vi "find frequency.vi"(9 "target frequency":dbl format="%.2f") -> (1 "Min":bool, 2 "Max":bool, 3 "ClockDivisor":i32, 4 "Frequency":dbl format="%.2f", 5 "FreqDivisor":i32, 6 "Clock Source":string)   [LabVIEW 2021]
panel:
  out "MinimumFreqOut freq at 48 MHz":dbl format="%.2f"
  out "Minimum FreqOut freq at 750k":dbl format="%.2f"
  in  "value, factor1, factor2":i32[][](array[numeric])=array65536x3[196608 elements]
  # "constant array of values"
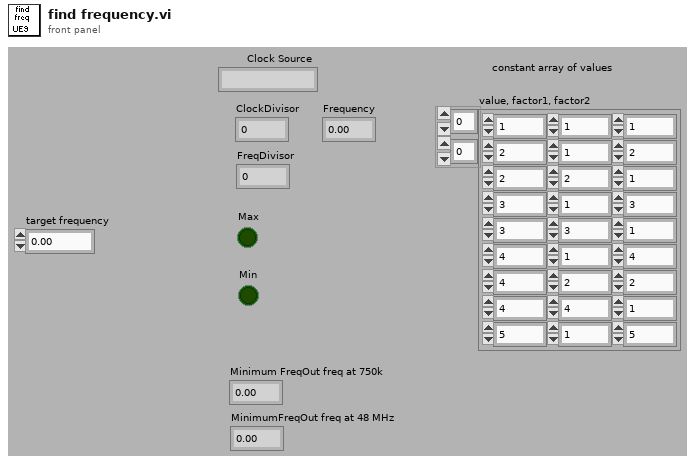
[diagram p1: front panel]
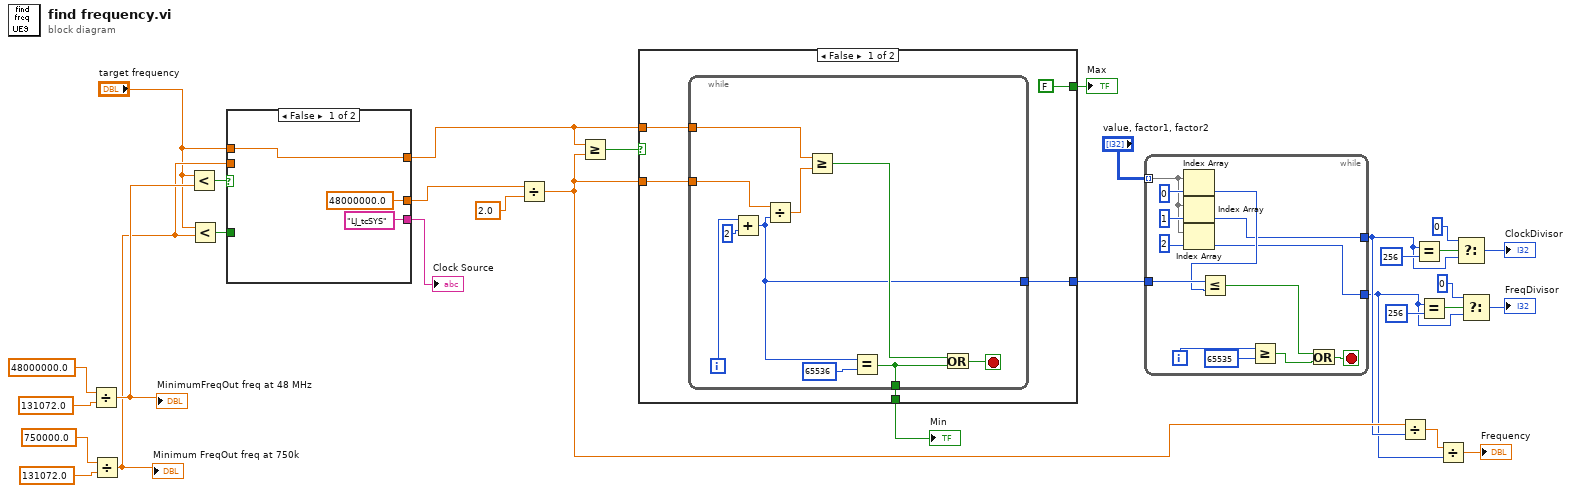
[diagram p0: block diagram]
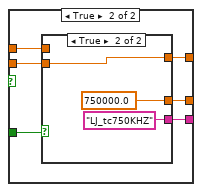
[diagram p2: hidden frame]
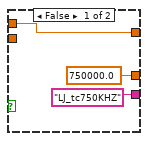
[diagram p3: hidden frame]
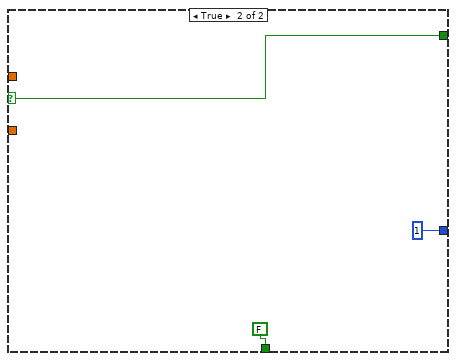
[diagram p4: hidden frame]
diagram:
  n1 = Divide(x=48000000.0, y=131072.0) -> (x/y=w6:dbl)
  "MinimumFreqOut freq at 48 MHz" <- w6
  n2 = Divide(x=750000.0, y=131072.0) -> (x/y=w5:dbl)
  "Minimum FreqOut freq at 750k" <- w5
  n3 = Less?(x="target frequency", y=w6) -> (x < y?=w12:bool)
  n4 = Less?(x="target frequency", y=w5) -> (x < y?=w11:bool)
  n5 = case shown="False" w12 {
    tunnel: w11 -> [_ w40]
    tunnel: ["LJ_tcSYS" w39] -> w1
    tunnel: [48000000.0 w38] -> w2
    tunnel: w5 -> [_ w37]
    tunnel: "target frequency" -> [w33 w36]
    tunnel: [w33 w35] -> w3
    frame False {
    }
    frame True {
      n6 = case shown="True" w40 {
        tunnel: ["LJ_tc750KHZ" "LJ_tc750KHZ"] -> w39
        tunnel: [750000.0 750000.0] -> w38
        tunnel: w37 -> [_ w45]
        tunnel: [w43 w45] -> w35
        tunnel: w36 -> [w43 _]
        frame False {
        }
        frame True {
        }
      }
    }
  }
  "Clock Source" <- w1
  n7 = Divide(x=w2, y=2.0) -> (x/y=w17:dbl)
  n8 = Greater Or Equal?(x=w3, y=w17) -> (x >= y?=w31:bool)
  n9 = case shown="False" w31 {
    selector: w31 -> [_ w64]
    tunnel: w17 -> [w51 _]
    tunnel: w3 -> [w50 _]
    tunnel: [w49 FALSE] -> w27
    tunnel: [FALSE w64] -> w30
    tunnel: [w47 1] -> w25
    frame False {
      n10 = while {
        tunnel: [w52] -> w47
        tunnel: [w53] -> w49
        tunnel: w50 -> [w57]
        tunnel: w51 -> [w61]
        i -> [w60]
        stop <- w56 stop-if-true
        n11 = Add(x=w60, y=2) -> (x+y=w52:i32)
        n12 = Divide(x=w61, y=w52) -> (x/y=w58:dbl)
        n13 = Greater Or Equal?(x=w57, y=w58) -> (x >= y?=w55:bool)
        n14 = Equal?(x=w52, y=65536) -> (x = y?=w53:bool)
        n15 = Or(x=w55, y=w53) -> (x .or. y?=w56:bool)
      }
    }
    frame True {
    }
  }
  "Max" <- w30
  "Min" <- w27
  n16 = while {
    tunnel: [w66] -> w15
    tunnel: [w67] -> w16
    tunnel: w25 -> [w76]
    tunnel: "value, factor1, factor2" -> [w65] mode=indexing
    i -> [w73]
    stop <- w77 stop-if-true
    n17 = Index Array(array=w65, index=0 ("Index")) -> (element=w68:i32)
    n18 = Index Array(array=w65, index=1 ("Index")) -> (element=w67:i32)
    n19 = Index Array(array=w65, index=2 ("Index")) -> (element=w66:i32)
    n20 = Less Or Equal?(x=w76, y=w68) -> (x <= y?=w75:bool)
    n21 = Greater Or Equal?(x=w73, y=65535) -> (x >= y?=w74:bool)
    n22 = Or(x=w75, y=w74) -> (x .or. y?=w77:bool)
  }
  n23 = Divide(x=w17, y=w16) -> (x/y=w14:dbl)
  n24 = Equal?(x=w16, y=256) -> (x = y?=w23:bool)
  n25 = Equal?(x=w15, y=256) -> (x = y?=w22:bool)
  n26 = Divide(x=w14, y=w15) -> (x/y=→"Frequency":dbl)
  n27 = Select(t=0, s=w23, f=w16) -> (s? t:f=→"ClockDivisor":i32)
  n28 = Select(t=0, s=w22, f=w15) -> (s? t:f=→"FreqDivisor":i32)
